vi "Files_Get_Paths.vi"(8 "error in (no error)":errorcluster, 10 "EXPERT Path Selector":T11=enum."XML Saved", 11 "Variant":variant) -> (0 "error out":errorcluster caption="sortie d'erreur", 3 "Path":path)   [LabVIEW 2018]
doc: "This VI returns the PATH of the day for the data, with the naming convention :\nDATA_PATH\\yyyy\\data_yyyy_mm_dd\\yyyy_mm_dd"
uses:
  controls/EXPERT_Path_Selector.ctl
  controls/EXPERT_Inputs.ctl
  controls/DIGIT_5122_Inputs.ctl
  <instrlib>/niScope/Controls/niScope trigger source.ctl
  controls/HSDIO_6541_Inputs.ctl
  <instrlib>/niHSDIO/niHSDIO.llb/niHSDIO_ctl Trigger Source Values (Ring).ctl
  controls/SOFTWARE_Inputs.ctl
  controls/AO_6711_Inputs.ctl
  controls/AWG_5421_Inputs.ctl
  <instrlib>/niFgen/niFgen.llb/niFgen_ctl Trigger Source Values (Ring).ctl
  controls/XML_Inputs.ctl
panel:
  in  "EXPERT Inputs":T1={"DIGIT 5122 Inputs"={"Sample Rate"=10000.0, "Resource Name"="DIGIT_5122", "Channel Name"="0", "Trigger Source"="VAL_EXTERNAL", "Vertical Range"=10.0, "Trigger Level"=3.0}, "HSDIO 6541 Inputs"={"Resource Name"="HSDIO_6541", "Clock Rate"=1000000.0, "Trigger Source"="PFI0"}, "SOFTWARE Inputs"={"Application Directory"=path "D:/S.O.F.T.S/LABVIEW/PIL", "Software Version"="1.0.0", "Data Path"=path "D:/PIRENEA/DATA", "XML Path"=path "D:/PIRENEA/DATA", "XML File Filter"="*.xml", "XML Saved Path"=path "D:/PIRENEA/DATA/SAVED", "Excit Scripts Path"=path "D:/PIRENEA/EXCIT_SCRIPTS", "Excit Scripts File Filter"="*.txt", "Excit Waveforms Path"=path "D:/PIRENEA/EXCIT_WFMS", "Excit Waveforms File Filter"="*.bin", "Timing Scripts Path"=path "D:/PIRENEA/TIMING_SCRIPTS", "Timing Scripts File Filter"="*.txt", "Timing Waveforms Path"=path "D:/PIRENEA/TIMING_WFMS", "Timing Waveforms File Filter"="*.bin", "Trapping Waveforms Path"=path "D:/PIRENEA/TRAPPING_WFMS", "Trapping Waveforms File Filter"="*.bin"}, "AO 6711 Inputs"={"Physical Channels"="AO_6711/ao0:3", "Min Voltage"=-10.0, "Max Voltage"=10.0, "Trigger Source"="/AO_6711/PFI3", "Counter"="AO_6711/ctr0"}, "AWG 5421 Inputs"={"Resource Name"="AWG_5421", "Sample Rate"=10000000.0, "Trigger Type"=2, "Trigger Source"="PFI0", "Waveform Gain"=0.31, "Digital Filter ON"=TRUE}, "XML Inputs"={"Version Tag Name"="XML_Version", "Version String"="1.0"}} {"AWG 5421 Inputs"."Sample Rate" format="%.2p"; "AWG 5421 Inputs"."Trigger Type" items=["None", "Software Edge", "Digital Edge", "Digital Level"]; "AO 6711 Inputs"."Max Voltage" min=-10.0 max=10.0; "AO 6711 Inputs"."Min Voltage" min=-10.0 max=10.0; "HSDIO 6541 Inputs"."Clock Rate" format="%.2p"; "DIGIT 5122 Inputs"."Trigger Level" format="%.2f"; "DIGIT 5122 Inputs"."Vertical Range" format="%.2f"; "DIGIT 5122 Inputs"."Sample Rate" step=65535.0 format="%#_3p"}
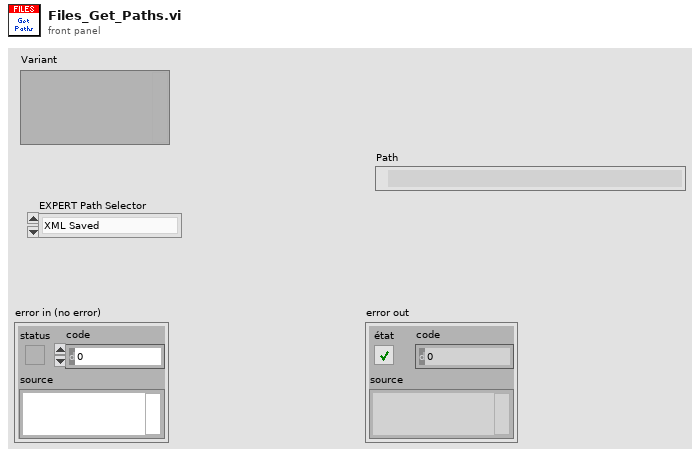
[diagram p1: front panel]
types:
  T1 = typedef "EXPERT_Inputs.ctl" = cluster{"DIGIT 5122 Inputs":T2, "HSDIO 6541 Inputs":T4, "SOFTWARE Inputs":T6, "AO 6711 Inputs":T7, "AWG 5421 Inputs":T8, "XML Inputs":T10}
  T2 = typedef "DIGIT_5122_Inputs.ctl" = cluster{"Sample Rate":dbl, "Resource Name":refnum<k15>, "Channel Name":string, "Trigger Source":T3, "Vertical Range":dbl, "Trigger Level":dbl}
  T3 = typedef "niScope trigger source.ctl" = string
  T4 = typedef "HSDIO_6541_Inputs.ctl" = cluster{"Resource Name":refnum<k15>, "Clock Rate":dbl, "Trigger Source":T5}
  T5 = typedef "niHSDIO_ctl Trigger Source Values (Ring).ctl" = string
  T6 = typedef "SOFTWARE_Inputs.ctl" = cluster{"Application Directory":path, "Software Version":string, "Data Path":path, "XML Path":path, "XML File Filter":string, "XML Saved Path":path, "Excit Scripts Path":path, "Excit Scripts File Filter":string, "Excit Waveforms Path":path, "Excit Waveforms File Filter":string, "Timing Scripts Path":path, "Timing Scripts File Filter":string, "Timing Waveforms Path":path, "Timing Waveforms File Filter":string, "Trapping Waveforms Path":path, "Trapping Waveforms File Filter":string}
  T7 = typedef "AO_6711_Inputs.ctl" = cluster{"Physical Channels":tag, "Min Voltage":dbl, "Max Voltage":dbl, "Trigger Source":tag, "Counter":tag}
  T8 = typedef "AWG_5421_Inputs.ctl" = cluster{"Resource Name":refnum<k15>, "Sample Rate":dbl, "Trigger Type":u16, "Trigger Source":T9, "Waveform Gain":dbl, "Digital Filter ON":bool}
  T9 = typedef "niFgen_ctl Trigger Source Values (Ring).ctl" = string
  T10 = typedef "XML_Inputs.ctl" = cluster{"Version Tag Name":string, "Version String":string}
  T11 = typedef "EXPERT_Path_Selector.ctl" = enum16{"Application", "Resources", "Data", "XML", "XML Saved", "Load Directory"}
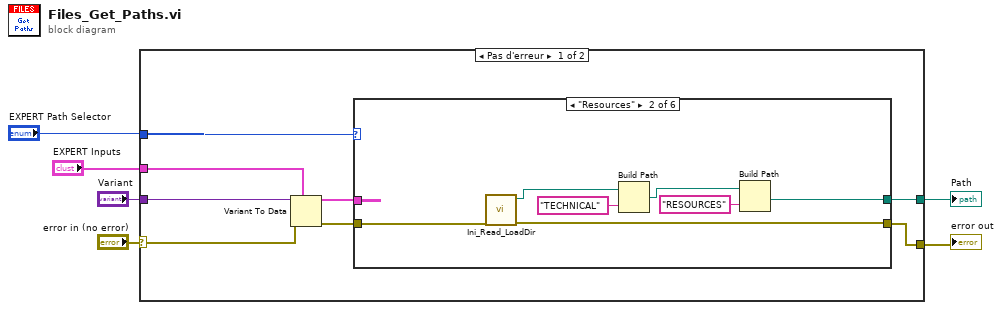
[diagram p0: block diagram]
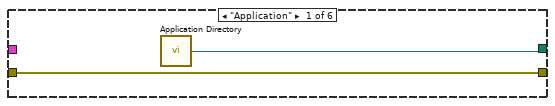
[diagram p2: hidden frame]
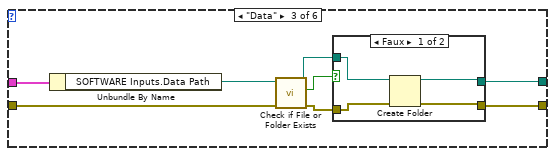
[diagram p3: hidden frame]
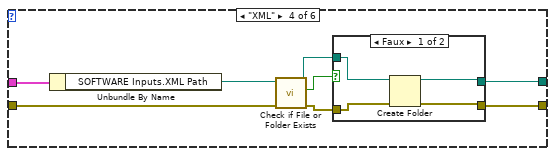
[diagram p5: hidden frame]
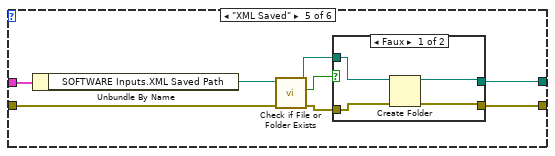
[diagram p7: hidden frame]
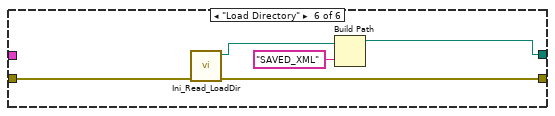
[diagram p9: hidden frame]
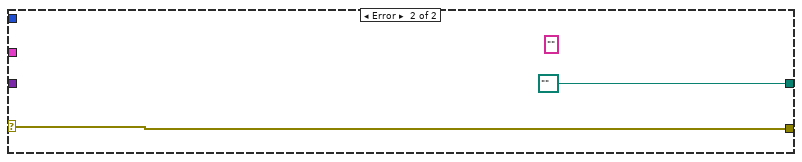
[diagram p10: hidden frame]
diagram:
  n1 = case shown="Pas d'erreur" "error in (no error)" {
    selector: "error in (no error)" -> [w8 w72]
    tunnel: [w10 w72] -> w5
    tunnel: "Variant" -> [w9 _]
    tunnel: "EXPERT Path Selector" -> [w13 _]
    tunnel: [w12 path "" ("Data Path")] -> w3
    tunnel: "EXPERT Inputs" -> [w7 _]
    frame No Error {
      n2 = Variant To Data(error in=w8, type=w7, Variant=w9) -> (data=w14:T1, error out=w11:errorcluster)
      n3 = case shown="\"Resources\"" w13 {
        tunnel: w14 -> [_ _ w31 w45 w59 _]
        tunnel: [w15 w18 w25 w39 w53 w67] -> w12
        tunnel: w11 -> [w16 w21 w26 w40 w54 w70]
        tunnel: [w16 w20 w24 w38 w52 w68] -> w10
        frame "Application" {
          n4 = call <vilib>:"Application Directory.vi"() -> ("Application Directory"=w15:path)
        }
        frame "Resources" {
          n5 = call "Ini_Read_LoadDir.vi"("error in (no error)"=w21) -> ("error out"=w20:errorcluster, "Path"=w23:path)  [unwired: 9 in]
          n6 = Build Path(base path=w23, name or relative path="TECHNICAL" ("nom ou chemin relatif")) -> (appended path=w19:path)
          n7 = Build Path(base path=w19, name or relative path="RESOURCES" ("nom ou chemin relatif")) -> (appended path=w18:path)
        }
        frame "Data" {
          n8 = Unbundle By Name(w31) -> ("SOFTWARE Inputs.Data Path"=w27:path)
          n9 = call <vilib>:"Check if File or Folder Exists.vi"("error in (no error)"=w26, "path"=w27) -> ("error out"=w30:errorcluster, "file or folder exists?"=w29:bool, "dup path"=w28:path)  [unwired: 7 in]
          n10 = case shown="Faux" w29 {
            tunnel: w30 -> [w35 w37]
            tunnel: w28 -> [w34 w36]
            tunnel: [w32 w37] -> w24
            tunnel: [w33 w36] -> w25
            frame False {
              n11 = Create Folder(path (use dialog)=w34, error in=w35) -> (created path=w33:path, error out=w32:errorcluster)  [unwired: 1 in, 1 out]
            }
            frame True {
            }
          }
        }
        frame "XML" {
          n12 = Unbundle By Name(w45) -> ("SOFTWARE Inputs.XML Path"=w41:path)
          n13 = call <vilib>:"Check if File or Folder Exists.vi"("error in (no error)"=w40, "path"=w41) -> ("error out"=w44:errorcluster, "file or folder exists?"=w43:bool, "dup path"=w42:path)  [unwired: 7 in]
          n14 = case shown="Faux" w43 {
            tunnel: w44 -> [w49 w51]
            tunnel: w42 -> [w48 w50]
            tunnel: [w46 w51] -> w38
            tunnel: [w47 w50] -> w39
            frame False {
              n15 = Create Folder(path (use dialog)=w48, error in=w49) -> (created path=w47:path, error out=w46:errorcluster)  [unwired: 1 in, 1 out]
            }
            frame True {
            }
          }
        }
        frame "XML Saved" {
          n16 = Unbundle By Name(w59) -> ("SOFTWARE Inputs.XML Saved Path"=w55:path)
          n17 = call <vilib>:"Check if File or Folder Exists.vi"("error in (no error)"=w54, "path"=w55) -> ("error out"=w58:errorcluster, "file or folder exists?"=w57:bool, "dup path"=w56:path)  [unwired: 7 in]
          n18 = case shown="Faux" w57 {
            tunnel: w58 -> [w63 w65]
            tunnel: w56 -> [w62 w64]
            tunnel: [w60 w65] -> w52
            tunnel: [w61 w64] -> w53
            frame False {
              n19 = Create Folder(path (use dialog)=w62, error in=w63) -> (created path=w61:path, error out=w60:errorcluster)  [unwired: 1 in, 1 out]
            }
            frame True {
            }
          }
        }
        frame "Load Directory" {
          n20 = call "Ini_Read_LoadDir.vi"("error in (no error)"=w70) -> ("error out"=w68:errorcluster, "Path"=w69:path)  [unwired: 9 in]
          n21 = Build Path(base path=w69, name or relative path="SAVED_XML" ("nom ou chemin relatif")) -> (appended path=w67:path)
        }
      }
    }
    frame Error {
      (unwired) "" ("XML File Filter")
    }
  }
  "error out" <- w5
  "Path" <- w3
